vi "ast_db_list.vi"() -> (3 "db":refnum<k1>)   [LabVIEW 2017]
uses:
  ql2proto/ql2proto_term_type.ctl
  ast_reql_cache_action.ctl
  ql2proto/ql2proto_term_type_encode.vi
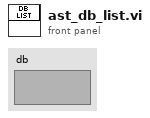
[diagram p1: front panel]
types:
  T1 = typedef "ast_reql_cache_action.ctl" = enum8{"null", "new", "get", "set", "pop"}
  T2 = typedef "ql2proto_term_type.ctl" = enum8{"DATUM", "MAKE_ARRAY", "MAKE_OBJ", "VAR", "JAVASCRIPT", "UUID", "HTTP", "ERROR", "IMPLICIT_VAR", "DB", "TABLE", "GET", "GET_ALL", "EQ", "NE", "LT", "LE", "GT", "GE", "NOT", "ADD", "SUB", "MUL", "DIV", "MOD", "FLOOR", "CEIL", "ROUND", "APPEND", "PREPEND", "DIFFERENCE", "SET_INSERT", "SET_INTERSECTION", "SET_UNION", "SET_DIFFERENCE", "SLICE", "SKIP", "LIMIT", "OFFSETS_OF", "CONTAINS", "GET_FIELD", "KEYS", "VALUES", "OBJECT", "HAS_FIELDS", "WITH_FIELDS", "PLUCK", "WITHOUT", "MERGE", "BETWEEN_DEPRECATED", "BETWEEN", "REDUCE", "MAP", "FOLD", "FILTER", "CONCAT_MAP", "ORDER_BY", "DISTINCT", "COUNT", "IS_EMPTY", "UNION", "NTH", "BRACKET", "INNER_JOIN", "OUTER_JOIN", "EQ_JOIN", "ZIP", "RANGE", "INSERT_AT", "DELETE_AT", "CHANGE_AT", "SPLICE_AT", "COERCE_TO", "TYPE_OF", "UPDATE", "DELETE", "REPLACE", "INSERT", "DB_CREATE", "DB_DROP", "DB_LIST", "TABLE_CREATE", "TABLE_DROP", "TABLE_LIST", "CONFIG", "STATUS", "WAIT", "RECONFIGURE", "REBALANCE", "SYNC", "GRANT", "INDEX_CREATE", "INDEX_DROP", "INDEX_LIST", "INDEX_STATUS", "INDEX_WAIT", "INDEX_RENAME", "SET_WRITE_HOOK", "GET_WRITE_HOOK", "FUNCALL", "BRANCH", "OR", "AND", "FOR_EACH", "FUNC", "ASC", "DESC", "INFO", "MATCH", "UPCASE", "DOWNCASE", "SAMPLE", "DEFAULT", "JSON", "ISO8601", "TO_ISO8601", "EPOCH_TIME", "TO_EPOCH_TIME", "NOW", "IN_TIMEZONE", "DURING", "DATE", "TIME_OF_DAY", "TIMEZONE", "YEAR", "MONTH", "DAY", "DAY_OF_WEEK", "DAY_OF_YEAR", "HOURS", "MINUTES", "SECONDS", "TIME", "MONDAY", "TUESDAY", "WEDNESDAY", "THURSDAY", "FRIDAY", "SATURDAY", "SUNDAY", "JANUARY", "FEBRUARY", "MARCH", "APRIL", "MAY", "JUNE", "JULY", "AUGUST", "SEPTEMBER", "OCTOBER", "NOVEMBER", "DECEMBER", "LITERAL", "GROUP", "SUM", "AVG", "MIN", "MAX", "SPLIT", "UNGROUP", "RANDOM", "CHANGES", "ARGS", "BINARY", "GEOJSON", "TO_GEOJSON", "POINT", "LINE", "POLYGON", "DISTANCE", "INTERSECTS", "INCLUDES", "CIRCLE", "GET_INTERSECTING", "FILL", "GET_NEAREST", "POLYGON_SUB", "TO_JSON_STRING", "MINVAL", "MAXVAL", "BIT_AND", "BIT_OR", "BIT_XOR", "BIT_NOT", "BIT_SAL", "BIT_SAR", "invalid"}
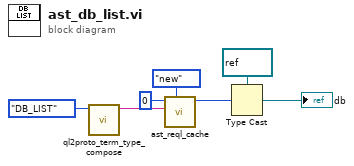
[diagram p0: block diagram]
diagram:
  w2 = refnum<k1> refnum items=["db"] ("db")
  n1 = call "ql2proto_term_type_compose.vi"("term_type"=ql2proto_term_type."DB_LIST") -> ("query"=w5:string)  [unwired: 10 in]
  n2 = call "ast_reql_cache.vi"("action"=ast_reql_cache_action."new", "query in"=w5, "reql_id in"=u32 0 ("query_id in")) -> ("reql_id out"=w3:u32)  [unwired: 6 in, 2 out]
  n3 = Type Cast(type=w2, x=w3) -> (*(type *) &x=→"db":refnum<k1>)
